vi "Tag Names 2.vi"(11 "?":T1={"State"=enum."Idle", "Start Time"=timestamp(0 s since 1904-01-01), "Current Time"=timestamp(0 s since 1904-01-01), "First Iteration"=FALSE, "Process Name"="", "Output Error"=FALSE, "Log Started"=FALSE, "Cycle Period"=50.0, "Configuration"={"Valve Settings"={"D-O Settings"={"DAQmx Task Name"="", "Output Channel"=0, "Output Channel Names"=[]}, "VICI Electronic Actuator"={"VISA resource name"="", "Mode"=enum."Two Positions With Stops", "Simulated"=FALSE}}, "Valve Type"=enum."Digital Output Valve", "Time On (Sec)"=0.0, "Time Off (Sec)"=0.0, "Run?"=FALSE}, "Data"={"D-O State"=enum."Off"}} {"Configuration"."Valve Settings"."D-O Settings"."Output Channel" items=["Choose a Channel"]}) -> (1 "output cluster":cluster{string[], string[]}, 2 "All Boolean Tags":string[](array[string]), 3 "All  Numeric Tags":string[](array[string]))   [LabVIEW 2018]
uses:
  State Cluster.ctl
  State Enum.ctl
  Valve Clusters.ctl
  D-O Module Settings Cluster.ctl
  D-O Device Settings Cluster.ctl
  VICI Electronic Actuator/VICI Electronic Actuator Settings.ctl
  D-O Module Engine.lvlib
  D-O Module.lvlib
  DIO Valve/VICI Electronic Actuator.lvlib
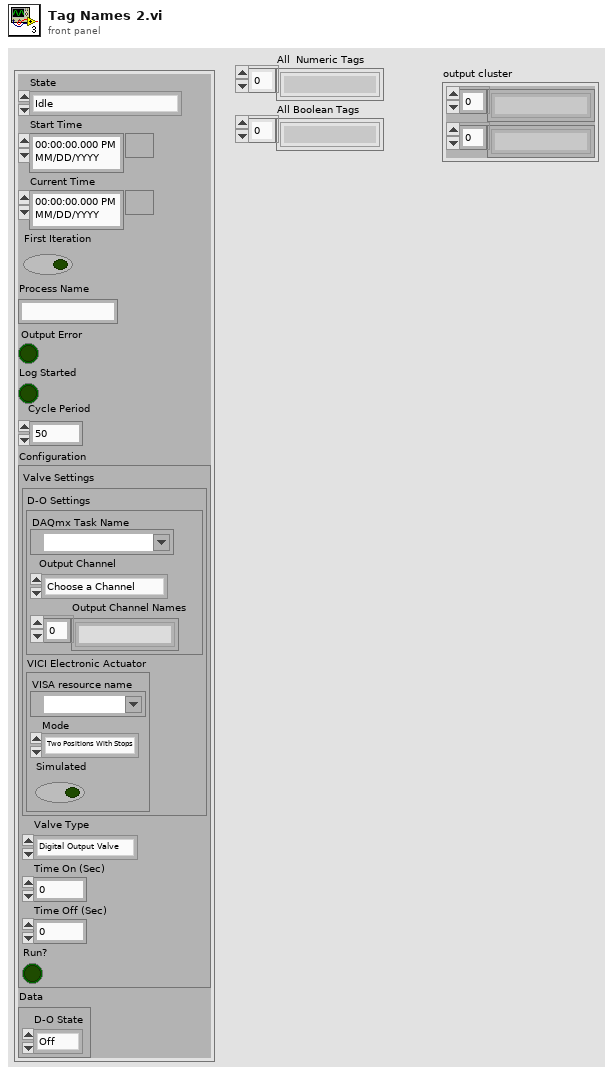
[diagram p1: front panel]
types:
  T1 = typedef "D-O Module.lvlib/D-O Module Engine.lvlib/State Cluster.ctl" = cluster{"State":T2, "Start Time":timestamp, "Current Time":timestamp, "First Iteration":bool, "Process Name":string, "Output Error":bool, "Log Started":bool, "Cycle Period":dbl, "Configuration":T3, "Data":cluster{"D-O State":enum16{"Off", "On", "Not Initialized"}}}
  T2 = typedef "D-O Module.lvlib/D-O Module Engine.lvlib/State Enum.ctl" = enum16{"Measuring", "Idle", "Paused"}
  T3 = typedef "D-O Module.lvlib/Valve Clusters.ctl" = cluster{"Valve Settings":T4, "Valve Type":enum16{"Default", "Digital Output Valve", "VICI Electronic Actuator"}, "Time On (Sec)":dbl, "Time Off (Sec)":dbl, "Run?":bool}
  T4 = typedef "D-O Module.lvlib/D-O Module Settings Cluster.ctl" = cluster{"D-O Settings":T5, "VICI Electronic Actuator":T6}
  T5 = typedef "D-O Module.lvlib/D-O Device Settings Cluster.ctl" = cluster{"DAQmx Task Name":refnum<k21>, "Output Channel":u16, "Output Channel Names":string[]}
  T6 = typedef "VICI Electronic Actuator.lvlib/VICI Electronic Actuator Settings.ctl" = cluster{"VISA resource name":refnum<visa-resource-name>, "Mode":enum16{"Two Positions With Stops", "Two Positions Without Stops", "Mutiposition"}, "Simulated":bool}
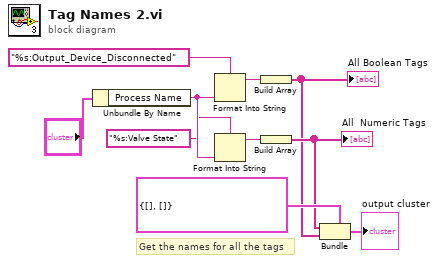
[diagram p0: block diagram]
diagram:
  # "Get the names for all the tags"
  n1 = Unbundle By Name("?") -> ("Process Name"=w9:string)
  n2 = Format Into String(format string="%s:Output_Device_Disconnected", w9) -> (resulting string=w4:string)  [unwired: 2 in, 1 out]
  n3 = Format Into String(format string="%s:Valve State", w9) -> (resulting string=w5:string)  [unwired: 2 in, 1 out]
  n4 = Build Array(w4) -> (w2:string[])
  "All Boolean Tags" <- w2
  n5 = Build Array(w5) -> (w3:string[])
  "All  Numeric Tags" <- w3
  n6 = Bundle(cluster=cluster{string[], string[]} {[], []}, w3, w2) -> (→"output cluster":cluster{string[], string[]})
